vi "Edit Team in Info.vi"(8 "Team GUID":i32, 9 "New Team Name":string, 10 "New Team Number":dbl, 11 "Team Info in":T1) -> (1 "Error String":string, 2 "Team Edited?":bool, 3 "Team Info out":T1)   [LabVIEW 2013]
uses:
  Team Data Array2.ctl
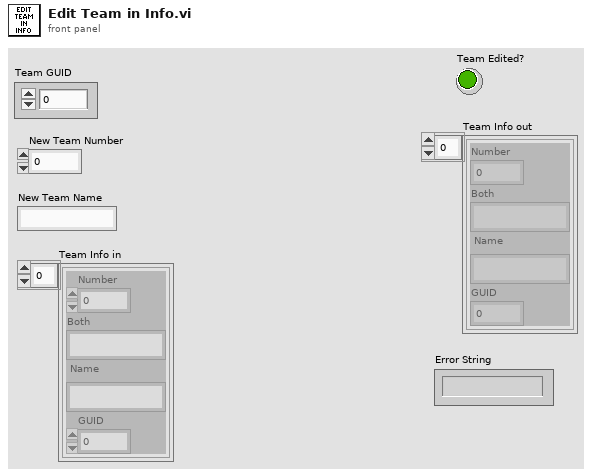
[diagram p1: front panel]
types:
  T1 = typedef "Team Data Array2.ctl" = cluster{"Number":u16, "Both":string, "Name":string, "GUID":u16}[]
  T2 = cluster{"[0]":cluster{"Number":u16, "Both":string, "Name":string, "GUID":u16}}
  T3 = cluster{"Number":u16, "Both":string, "Name":string, "GUID":u16}
  T4 = cluster{"Number":u16, "Both":string, "Name":string, "GUID":u16}[]
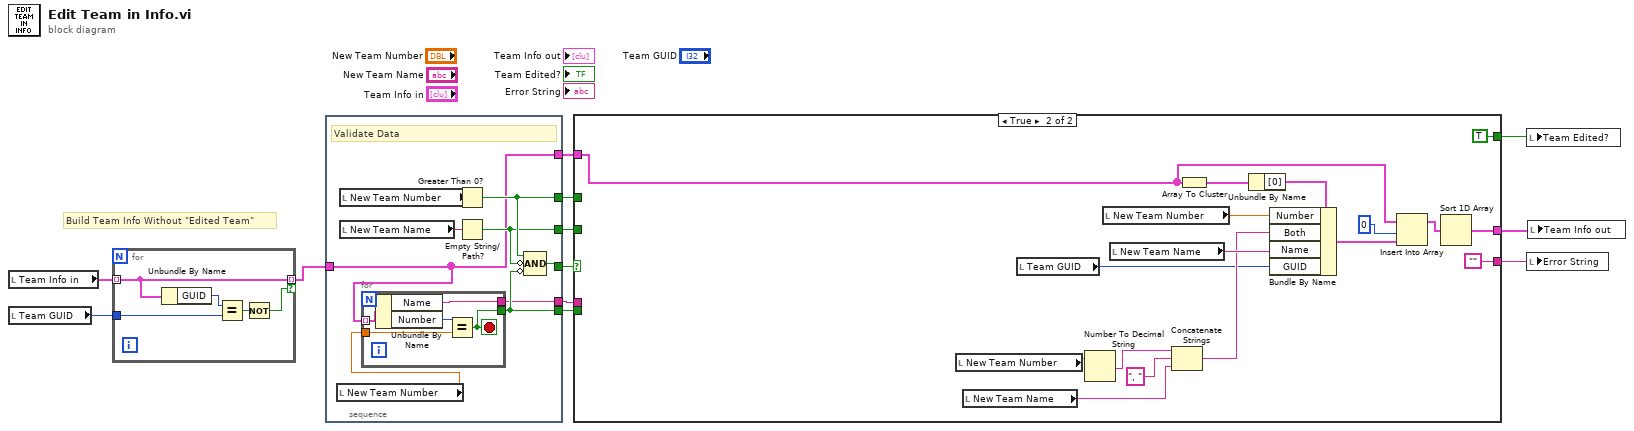
[diagram p0: block diagram]
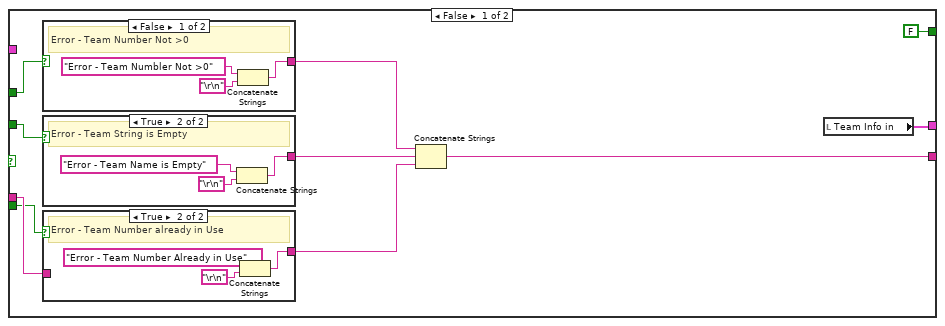
[diagram p2: hidden frame]
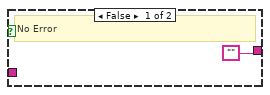
[diagram p3: hidden frame]
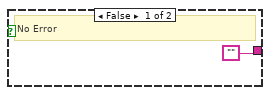
[diagram p4: hidden frame]
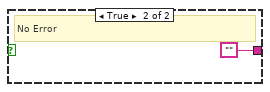
[diagram p5: hidden frame]
diagram:
  # "Build Team Info Without \"Edited Team\""
  n1 = local read "Team Info in"() -> (w4:T1)
  n2 = local read "Team GUID"() -> (w3:i32)
  n3 = for {
    tunnel: w4 -> [w15] mode=indexing
    tunnel: w3 -> [w16]
    tunnel: [w15] -> w2 mode=indexing if=w13
    n4 = Unbundle By Name(w15) -> ("GUID"=w17:u16)
    n5 = Equal?(x=w17, y=w16) -> (x = y?=w14:bool)
    n6 = Not(x=w14) -> (.not. x?=w13:bool)
  }
  n7 = stacked-sequence {
    tunnel: [w23] -> w12
    tunnel: [w22] -> w11
    tunnel: [w21] -> w10
    tunnel: [w20] -> w9
    tunnel: [w19] -> w8
    tunnel: w2 -> [w18]
    tunnel: [w18] -> w1
    frame #0 {
      # "Validate Data"
      n8 = local read "New Team Number"() -> (w24:dbl)
      n9 = local read "New Team Number"() -> (w26:dbl)
      n10 = local read "New Team Name"() -> (w25:string)
      n11 = for {
        tunnel: w18 -> [w31] mode=indexing
        tunnel: w24 -> [w29]
        tunnel: [w28] -> w20
        tunnel: [w27] -> w19
        stop <- w28 stop-if-true
        n12 = Unbundle By Name(w31) -> ("Name"=w27:string, "Number"=w30:u16)
        n13 = Equal?(x=w30, y=w29) -> (x = y?=w28:bool)
      }
      n14 = Greater Than 0?(x=w26) -> (x > 0?=w22:bool)
      n15 = Empty String/Path?(string/path=w25) -> (empty?=w21:bool)
      n16 = Compound Arithmetic op=AND(w22, invert w21, invert w20) -> (w23:bool)
    }
  }
  n17 = case shown="True" w12 {
    tunnel: [FALSE TRUE] -> w7
    tunnel: w11 -> [w40 _]
    tunnel: w10 -> [w39 _]
    tunnel: w9 -> [w37 _]
    tunnel: w8 -> [w38 _]
    tunnel: [w33 ""] -> w6
    tunnel: [w32 w56] -> w5
    tunnel: w1 -> [_ w54]
    frame False {
      n18 = case shown="False" w40 {
        tunnel: [w50 ""] -> w36
        frame False {
          # "Error - Team Number Not >0"
          n19 = Concatenate Strings("Error - Team Numbler Not >0", "\r\n") -> (w50:string)
        }
        frame True {
          # "No Error"
        }
      }
      n20 = case shown="True" w39 {
        tunnel: ["" w47] -> w35
        frame False {
          # "No Error"
        }
        frame True {
          # "Error - Team String is Empty"
          n21 = Concatenate Strings("Error - Team Name is Empty", "\r\n") -> (w47:string)
        }
      }
      n22 = case shown="True" w37 {
        tunnel: ["" w43] -> w34
        tunnel: w38 -> [_ _]
        frame False {
          # "No Error"
        }
        frame True {
          # "Error - Team Number already in Use"
          n23 = Concatenate Strings("Error - Team Number Already in Use", "\r\n") -> (w43:string)
        }
      }
      n24 = Concatenate Strings(w36, w35, w34) -> (w33:string)
      n25 = local read "Team Info in"() -> (w32:T1)
    }
    frame True {
      n26 = local read "New Team Number"() -> (w64:dbl)
      n27 = local read "New Team Name"() -> (w61:string)
      n28 = local read "Team GUID"() -> (w55:i32)
      n29 = Number To Decimal String(number=w64) -> (decimal integer string=w62:string)  [unwired: 1 in]
      n30 = local read "New Team Number"() -> (w66:dbl)
      n31 = local read "New Team Name"() -> (w65:string)
      n32 = Concatenate Strings(w62, ", ", w61) -> (w60:string)
      n33 = Array To Cluster(array=w54) -> (cluster=w68:T2)
      n34 = Unbundle By Name(w68) -> ("[0]"=w67:T3)
      n35 = Bundle By Name(cluster=w67, "Number"=w66, "Both"=w60, "Name"=w65, "GUID"=w55) -> (w59:T3)
      n36 = Insert Into Array(array=w54, index=0, new element=w59) -> (w57:T4)
      n37 = Sort 1D Array(array=w57) -> (sorted array=w56:T4)
    }
  }
  n38 = local write "Team Edited?"(w7) -> ()
  n39 = local write "Error String"(w6) -> ()
  n40 = local write "Team Info out"(w5) -> ()
